vi "Spectrogram.vi"(0 "X":dbl[](array[numeric]), 1 "Intensity Graph ref":refnum<vi>, 5 "Fs (Hz)":dbl, 7 "freq binwidth (Hz)":dbl, 9 "time binwidth (s)":dbl) -> ()   [LabVIEW 2015]
uses:
  <vilib>/gmath/NI_Gmath.lvlib
panel:
  out "error out":errorcluster
  in  "error in (no error)":errorcluster
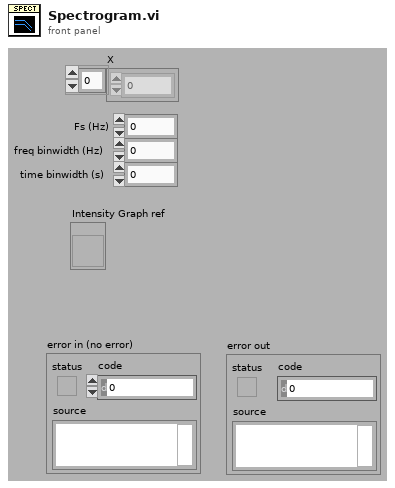
[diagram p1: front panel]
types:
  T1 = cluster{"force freq bins to power of 2?":bool, "exclude Nyquist frequency?":bool}
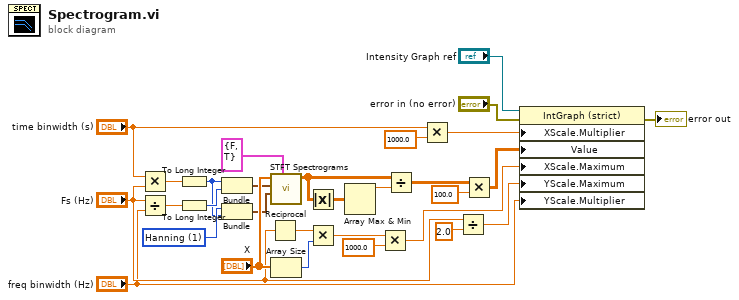
[diagram p0: block diagram]
diagram:
  w9 = u32 1 items=["Rectangle"=0, "Hanning"=1, "Hamming"=2, "Blackman-Harris"=3, "Exact Blackman"=4, "Blackman"=5, "Flat Top"=6, "4 Term B-Harris "=7, "7 Term B-Harris"=8, "Low Sidelobe"=9, "Blackman Nuttall"=11, "Triangle"=30, "Gaussian"=62] ("type")
  n1 = Multiply(x="time binwidth (s)", y="Fs (Hz)") -> (x*y=w15:dbl)
  n2 = Divide(x="Fs (Hz)", y="freq binwidth (Hz)") -> (x/y=w22:dbl)
  n3 = To Long Integer(number=w15) -> (32bit integer=w8:i32)
  n4 = To Long Integer(number=w22) -> (32bit integer=w21:i32)
  n5 = Bundle(w8, w21) -> (w20:cluster{i32, i32})  [unwired: 1 in]
  n6 = Bundle("type"=w9, w8) -> (w7:cluster{"type":u32, i32})  [unwired: 1 in]
  n7 = Reciprocal(x="Fs (Hz)") -> (1/x=w25:dbl)
  n8 = call <vilib>:"STFT Spectrograms.vi"("time-freq config"=T1 {"force freq bins to power of 2?"=FALSE, "exclude Nyquist frequency?"=TRUE}, "window info"=w7, "time-freq sampling info"=w20, "X"="X") -> ("STFT Spectrogram {X}"=w17:dbl[][])  [unwired: 6 in, 1 out]
  n9 = Array Size(array="X") -> (size(s)=w24:i32)
  n10 = Absolute Value(x=w17) -> (abs(x)=w30:dbl[][])
  n11 = Multiply(x=w25, y=w24) -> (x*y=w14:dbl)
  n12 = Array Max & Min(array=w30) -> (max value=w29:dbl)  [unwired: 3 out]
  n13 = Multiply(x=w14, y=1000.0) -> (x*y=w13:dbl)
  n14 = Divide(x=w17, y=w29) -> (x/y=w28:dbl[][])
  n15 = Multiply(x="time binwidth (s)", y=1000.0) -> (x*y=w6:dbl)
  n16 = Divide(x="Fs (Hz)", y=2.0) -> (x/y=w3:dbl)
  n17 = Multiply(x=w28, y=100.0) -> (x*y=w5:dbl[][])
  n18 = property class="IntGraph (strict)"(reference="Intensity Graph ref", error in="error in (no error)", "XScale.Multiplier"=w6, "Value"=w5, "XScale.Maximum"=w13, "YScale.Maximum"=w3, "YScale.Multiplier"="freq binwidth (Hz)") -> (error out=→"error out":errorcluster)  [unwired: 1 out]
